vi "Make 1D marginal PDF_V_PN.vi"(2 "dV":dbl, 3 "dU*":dbl, 4 "V*min":dbl, 5 "2D PDF (U,V)":dbl[][](array[numeric])) -> (0 "1D marginal PDF (V)":dbl[](array[numeric]), 1 "V bin centre vals":dbl[](array[numeric]))   [LabVIEW 2010]
panel:
  out "1D marginal PDF (V)":cluster{dbl[], dbl[]}(graph)
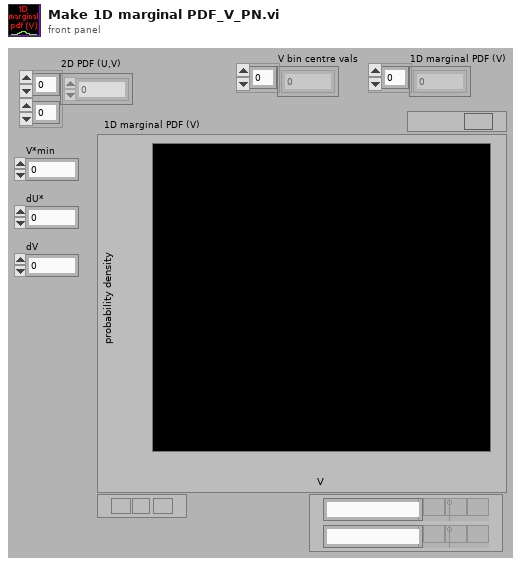
[diagram p1: front panel]
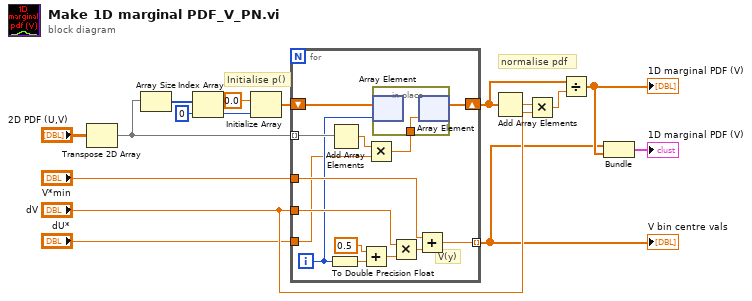
[diagram p0: block diagram]
diagram:
  # "normalise pdf"
  # "Initialise p()"
  n1 = Transpose 2D Array(2D array="2D PDF (U,V)") -> (transposed array=w4:dbl[][])
  n2 = Array Size(array=w4) -> (size(s)=w7:i32[])
  n3 = Index Array(array=w7, index=0) -> (element=w5:i32)
  n4 = Initialize Array(0.0 ("element"), w5) -> (w15:dbl[])
  n5 = for {
    tunnel: "dU*" -> [w19]
    shift-right: [w17] -> w13
    shift-left: w15 -> [w21]
    tunnel: [w26] -> w1 mode=indexing
    tunnel: "V*min" -> [w25]
    tunnel: "dV" -> [w24]
    tunnel: w4 -> [w23] mode=indexing
    i -> [w22]
    # "y"
    # "V(y)"
    n6 = To Double Precision Float(number=w22) -> (double precision float=w29:dbl)
    n7 = Add Array Elements(numeric array=w23) -> (sum=w20:dbl)
    n8 = Add(x=0.5, y=w29) -> (x+y=w28:dbl)
    n9 = Multiply(x=w20, y=w19) -> (x*y=w18:dbl)
    n10 = in-place {
      in-place-border: w18 -> [w31]
      n11 = in-place-array #1(w21, w22) -> ()  [unwired: 1 out]
      n12 = in-place-array #1(w31) -> (w17:dbl[])  [unwired: 1 out]
    }
    n13 = Multiply(x=w24, y=w28) -> (x*y=w27:dbl)
    n14 = Add(x=w25, y=w27) -> (x+y=w26:dbl)
  }
  "V bin centre vals" <- w1
  n15 = Add Array Elements(numeric array=w13) -> (sum=w14:dbl)
  n16 = Multiply(x=w14, y="dV") -> (x*y=w12:dbl)
  n17 = Divide(x=w13, y=w12) -> (x/y=w10:dbl[])
  "1D marginal PDF (V)" <- w10
  n18 = Bundle(w1, w10) -> (→"1D marginal PDF (V)":cluster{dbl[], dbl[]})  [unwired: 1 out]
